vi "AnalogOutput Interface SquareSequence1.vi"(7 "Options":T2={"Waveform type"=enum."square", "Sample clock (Hz)"=100000.0}, 8 "Eventstring":string, 11 "Port index":i32) -> (1 "OutputRequest":T3)   [LabVIEW 2015]
doc: "Makes OutputRequest objects compatible with the AnalogOutput output driver for a sequence of sines.\n\nCurrently only does sine waves\n\nPort index: Port number assigned by the reservation system\nSine sequence: Array of clusters; each cluster describes one sine (they get appended together)\n Frequency (Hz): Frequency of sine wave\n Amplitude (V): Peak amplitude in V\n Duration (ms): Duration of tone\nEventstring: String to send w/ timestamp, or empty/unwired for no timestamp\nOptions:\n Waveform type: Only one choice: \"sine\"\n Sample clock (Hz): Rate to sample the signal at"
uses:
  Typedefs/OutputRequest.ctl
  Typedefs/AnalogOutput_SquareSequence.ctl
panel:
  in  "Square sequence":T1(array[cluster])
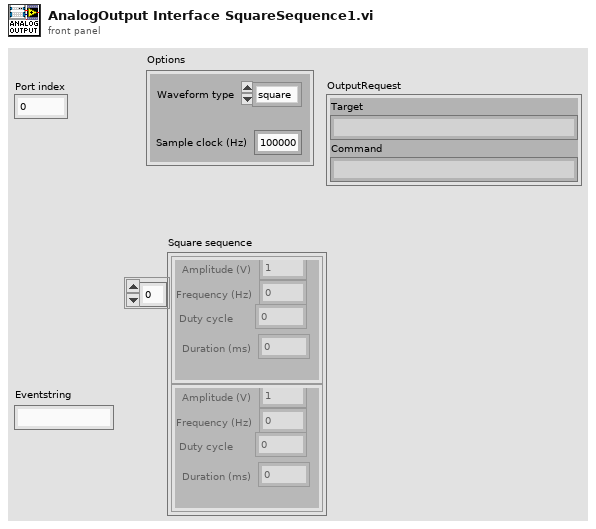
[diagram p1: front panel]
types:
  T1 = cluster{"Frequency (Hz)":dbl, "Duty cycle":dbl, "Amplitude (V)":dbl, "Duration (ms) ":dbl}[]
  T2 = cluster{"Waveform type":enum16{"square"}, "Sample clock (Hz)":dbl}
  T3 = typedef "OutputRequest.ctl" = cluster{"Target":string, "Command":string}
  T4 = typedef "AnalogOutput_SquareSequence.ctl" = cluster{"Frequency (Hz)":dbl, "Duty Cycle":dbl, "Duration (ms)":dbl, "Sample clock (Hz)":dbl, "Amplitude (V)":dbl}[]
  T5 = cluster{"Frequency (Hz)":dbl, "Duty Cycle":dbl, "Duration (ms)":dbl, "Sample clock (Hz)":dbl, "Amplitude (V)":dbl}
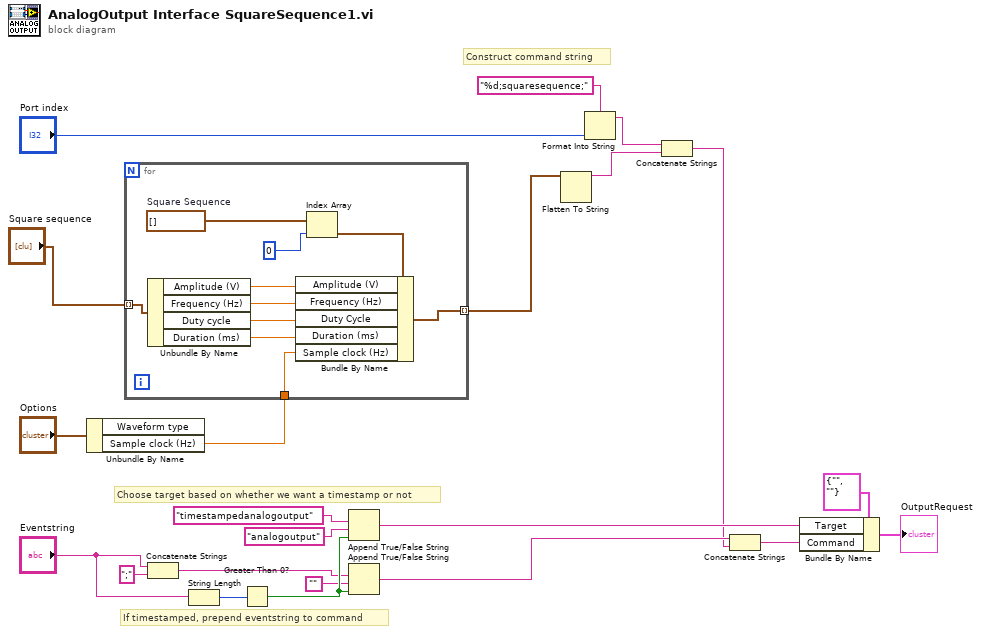
[diagram p0: block diagram]
diagram:
  # "Construct command string"
  # "If timestamped, prepend eventstring to command"
  # "Choose target based on whether we want a timestamp or not"
  n1 = Unbundle By Name("Options") -> ("Sample clock (Hz)"=w4:dbl)  [unwired: 1 out]
  n2 = for {
    tunnel: "Square sequence" -> [w32] mode=indexing
    tunnel: w4 -> [w25]
    tunnel: [w26] -> w3 mode=indexing
    w23 = T4 []  # Square Sequence
    n3 = Unbundle By Name(w32) -> ("Amplitude (V)"=w29:dbl, "Frequency (Hz)"=w28:dbl, "Duty cycle"=w27:dbl, "Duration (ms)"=w24:dbl)
    n4 = Index Array(array=w23, index=0) -> (element=w30:T5)
    n5 = Bundle By Name(cluster=w30, "Amplitude (V)"=w29, "Frequency (Hz)"=w28, "Duty Cycle"=w27, "Duration (ms)"=w24, "Sample clock (Hz)"=w25) -> (w26:T5)
  }
  n6 = Concatenate Strings("Eventstring", ";" ("string")) -> (w13:string)
  n7 = String Length(string="Eventstring") -> (length=w20:i32)
  n8 = Greater Than 0?(x=w20) -> (x > 0?=w14:bool)
  n9 = Append True/False String(1:w14, 2:"analogoutput" ("false string"), 3:"timestampedanalogoutput" ("true string")) -> (0:w17:string)  [unwired: 1 in]
  n10 = Append True/False String(1:w14, 2:"", 3:w13) -> (0:w10:string)  [unwired: 1 in]
  n11 = Flatten To String(anything=w3) -> (data string=w5:string)  [unwired: 3 in, 2 out]
  n12 = Format Into String(format string="%d;squaresequence;", "Port index") -> (resulting string=w6:string)  [unwired: 2 in, 1 out]
  n13 = Concatenate Strings(w6, w5) -> (w2:string)
  n14 = Concatenate Strings(w10, w2) -> (w11:string)
  n15 = Bundle By Name(cluster=T3 {"Target"="", "Command"=""} ("OutputRequest"), "Target"=w17, "Command"=w11) -> (→"OutputRequest":T3)
